vi "Get Media Type.vi"(8 "Error In":errorcluster, 11 "XBMC Ref":T1) -> (0 "Error Out":errorcluster, 2 "Media Type":T3, 3 "XBMC Ref":T1)   [LabVIEW 2013, in "LMH-Kodi.lvlib"]
doc: "Get the media type currently playing."
uses:
  LMH-Kodi.lvlib
  Private/Player/Type Defs/Media Type.ctl
  Private/Type Defs/XBMC Ref.ctl
  <vilib>/httpClient/ClientHandle.ctl
  Private/Type Defs/Error.ctl
  <vilib>/httpClient/LabVIEWHTTPClient.lvlib
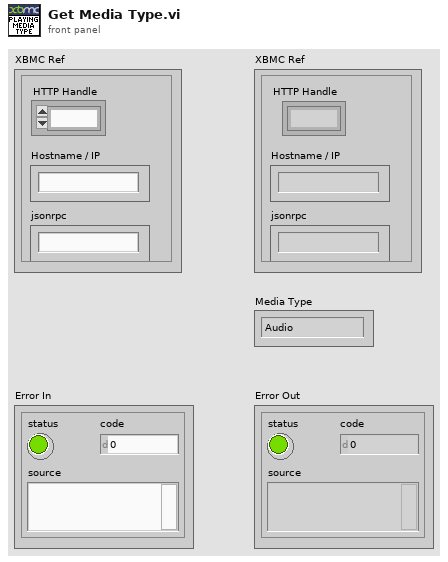
[diagram p1: front panel]
types:
  T1 = typedef "LMH-Kodi.lvlib/XBMC Ref.ctl" = cluster{"HTTP Handle":T2, "Hostname / IP":string, "jsonrpc":string}
  T2 = typedef "LabVIEWHTTPClient.lvlib/ClientHandle.ctl" = refnum<k1>
  T3 = typedef "LMH-Kodi.lvlib/Player.lvlib/Media Type.ctl" = enum8{"Audio", "Video", "Picture", "None", "Error"}
  T4 = typedef "LMH-Kodi.lvlib/Error.ctl" = enum16{"Unauthorized", "XBMC Error", "JSON Parse Error"}
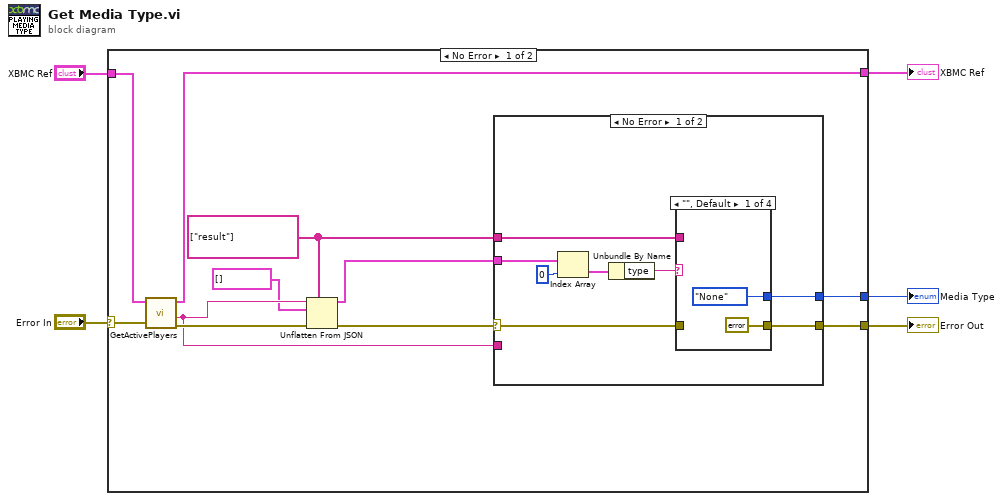
[diagram p0: block diagram]
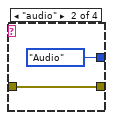
[diagram p2: hidden frame]
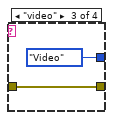
[diagram p3: hidden frame]
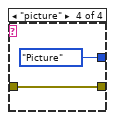
[diagram p4: hidden frame]
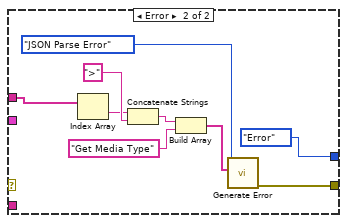
[diagram p5: hidden frame]
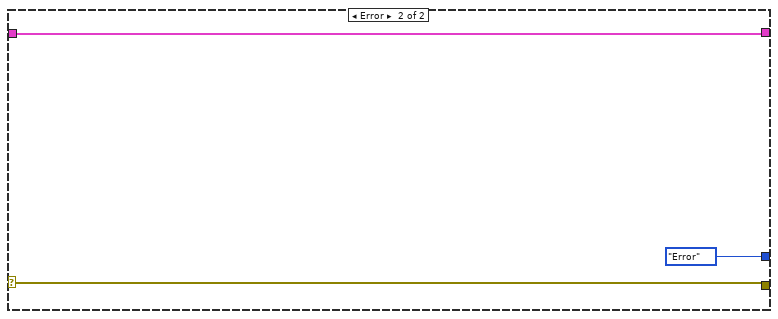
[diagram p6: hidden frame]
diagram:
  n1 = case shown="No Error" "Error In" {
    selector: "Error In" -> [w12 w44]
    tunnel: [w16 Media_Type."Error" ("Media Type")] -> w5
    tunnel: "XBMC Ref" -> [w15 w42]
    tunnel: [w14 w42] -> w3
    tunnel: [w13 w44] -> w2
    frame No Error {
      w11 = string[] ["result"] ("path")
      n2 = call "GetActivePlayers.vi"("Error In"=w12, "XBMC Ref"=w15) -> ("Error Out"=w10:errorcluster, "Response"=w8:string, "XBMC Ref"=w14:T1)  [unwired: 7 in]
      n3 = Unflatten From JSON(path=w11, JSON string=w8, type and defaults=cluster{"playerid":i32, "type":string}[] [], error in (no error)=w10) -> (value=w6:cluster{"playerid":i32, "type":string}[], error out=w9:errorcluster)  [unwired: 3 in]
      n4 = case shown="No Error" w9 {
        selector: w9 -> [w21 _]
        tunnel: [w24 Media_Type."Error" ("Media Type")] -> w16
        tunnel: [w23 w40] -> w13
        tunnel: w11 -> [w22 w33]
        tunnel: w8 -> [_ _]
        tunnel: w6 -> [w18 _]
        frame No Error {
          n5 = Index Array(array=w18, index=0) -> (element=w20:cluster{"playerid":i32, "type":string})
          n6 = Unbundle By Name(w20) -> ("type"=w17:string)
          n7 = case shown="\"\", Default" w17 {
            tunnel: [Media_Type."None" ("Media Type") Media_Type."Audio" ("Media Type") Media_Type."Video" ("Media Type") Media_Type."Picture" ("Media Type")] -> w24
            tunnel: [errorcluster {"status"=FALSE, "code"=0, "source"=""} ("error out") w27 w29 w31] -> w23
            tunnel: w21 -> [_ w27 w29 w31]
            tunnel: w22 -> [_ _ _ _]
            frame "", Default {
            }
            frame "audio" {
            }
            frame "video" {
            }
            frame "picture" {
            }
          }
        }
        frame Error {
          n8 = Index Array(array=w33) -> (element=w34:string)  [unwired: 1 in]
          n9 = Concatenate Strings(w34, ">" ("string")) -> (w38:string)
          n10 = Build Array(w38, "Get Media Type" ("element")) -> (w36:string[])
          n11 = call "Generate Error.vi"("Arguments"=w36, "Error"=Error."JSON Parse Error") -> ("Error Out"=w40:errorcluster)  [unwired: 9 in]
        }
      }
    }
    frame Error {
    }
  }
  "Error Out" <- w2
  "Media Type" <- w5
  "XBMC Ref" <- w3
